vi "Update Status.vi"(8 "error in (no error)":errorcluster, 10 "Status":string, 11 "UI Status in":refnum<class "UI Status.lvclass">) -> (0 "error out":errorcluster, 3 "UI Status out":refnum<class "UI Status.lvclass">)   [LabVIEW 2020, in "UI Status.lvlib" / "UI Status.lvclass"]
uses:
  UI Status.lvclass
  UI Status.lvclass/UI Status.ctl
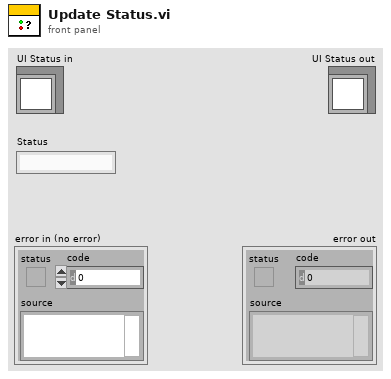
[diagram p1: front panel]
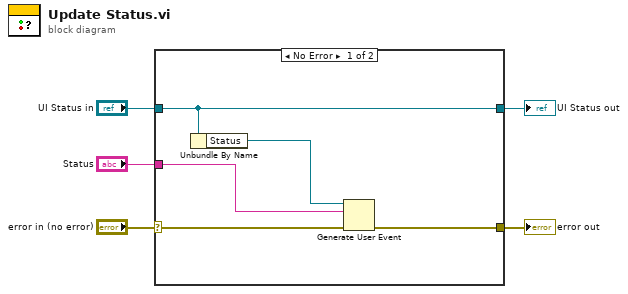
[diagram p0: block diagram]
diagram:
  n1 = case shown="No Error" "error in (no error)" {
    selector: "error in (no error)" -> [w9 w12]
    tunnel: [w8 w12] -> w4
    tunnel: [w10 w11] -> w2
    tunnel: "UI Status in" -> [w10 w11]
    tunnel: "Status" -> [w6 _]
    frame No Error {
      n2 = Unbundle By Name(w10) -> ("Status"=w7:refnum<user-event>)
      n3 = Generate User Event(user event=w7, event data cluster=w6, error in=w9) -> (error out=w8:errorcluster)  [unwired: 1 in, 1 out]
    }
    frame Error {
    }
  }
  "error out" <- w4
  "UI Status out" <- w2
